vi "authenticationsreader.vi"(1 "error (in)":errorcluster) -> (0 "error (out)":errorcluster)   [LabVIEW 2016]
doc: "Grab the .project8_authentications.json file in the home and read the AMQP credentials."
uses:
  global/AMQP_credentials.vi
panel:
  out "Path":path
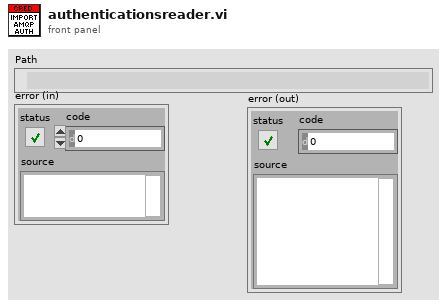
[diagram p1: front panel]
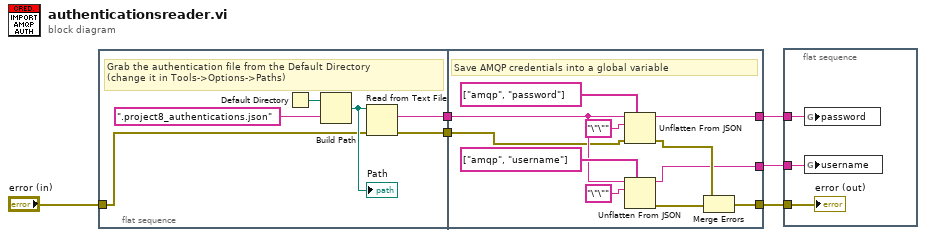
[diagram p0: block diagram]
diagram:
  n1 = flat-sequence {
    tunnel: [w9] -> w6
    tunnel: [w8] -> w5
    tunnel: "error (in)" -> [w7]
    tunnel: w6 -> [w19]
    tunnel: w5 -> [w18]
    tunnel: [w15] -> w2
    tunnel: [w14] -> w4
    tunnel: [w13] -> w3
    frame #0 {
      # "Grab the authentication file from the Default Directory\n(change it in Tools->Options->Paths)"
      n2 = Default Directory() -> (w10:path)
      n3 = Build Path(base path=w10, name or relative path=".project8_authentications.json") -> (appended path=w12:path)
      "Path" <- w12
      n4 = Read from Text File(file (use dialog)=w12, error in=w7) -> (text=w9:string, error out=w8:errorcluster)  [unwired: 2 in, 2 out]
    }
    frame #1 {
      # "Save AMQP credentials into a global variable"
      n5 = Unflatten From JSON(path=string[] ["amqp", "password"], JSON string=w19, type and defaults="\"\"", error in (no error)=w18) -> (value=w14:string, error out=w17:errorcluster)  [unwired: 3 in]
      n6 = Unflatten From JSON(path=string[] ["amqp", "username"], JSON string=w19, type and defaults="\"\"") -> (value=w13:string, error out=w16:errorcluster)  [unwired: 4 in]
      n7 = Merge Errors(w17, w16) -> (w15:errorcluster)
    }
  }
  n8 = flat-sequence {
    tunnel: w4 -> [w26]
    tunnel: w3 -> [w25]
    tunnel: w2 -> [w24]
    frame #0 {
      n9 = global write "AMQP_credentials.vi" "password"(w26) -> ()
      n10 = global write "AMQP_credentials.vi" "username"(w25) -> ()
      "error (out)" <- w24
    }
  }
